vi "main.vi"() -> ()   [LabVIEW 2023]
uses:
  <vilib>/Utility/error.llb/DialogType.ctl
panel:
  in  "Stop":bool
  out "error out":errorcluster
  in  "error in (no error)":errorcluster
  out "Output":string
  in  "Commands":string
  in  "Execute":bool
  # "Note:\n    - SOURce:VOLTage:DC <voltage> \n    - SOURce:CURRent:DC <voltage>\n    - MEASure:VOLTage:DC ? \n    - MEASure:CURRent:DC ?"
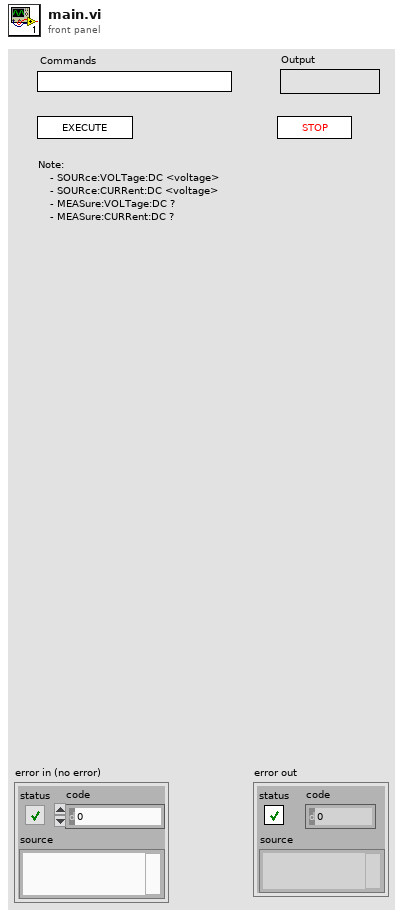
[diagram p1: front panel]
types:
  T1 = typedef "DialogType.ctl" = u16
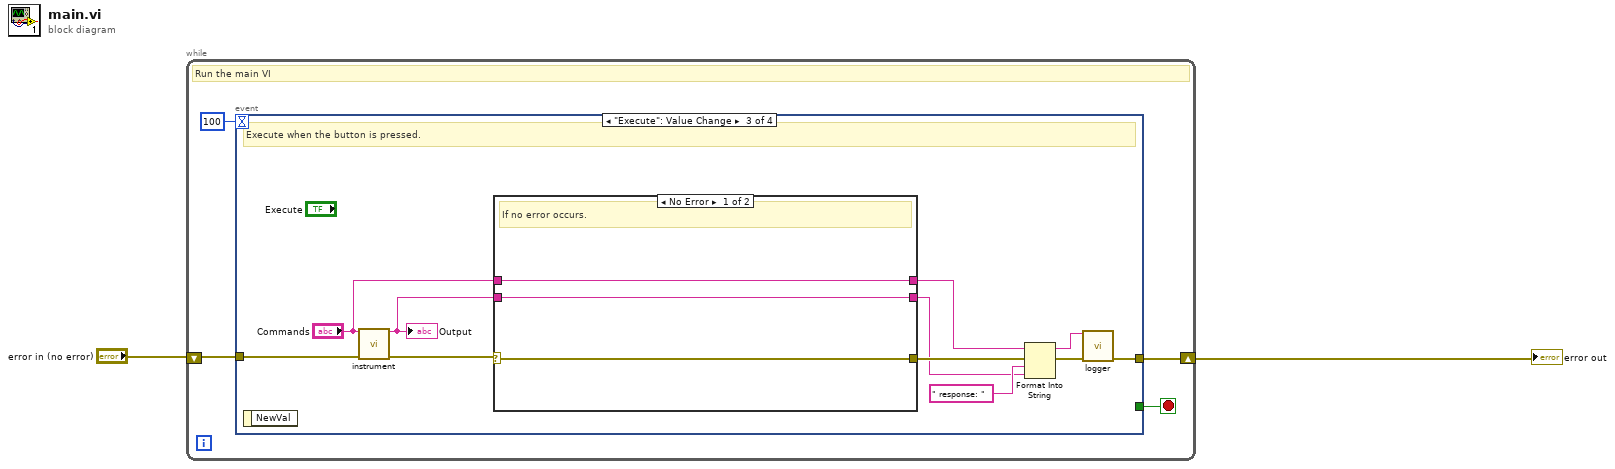
[diagram p0: block diagram]
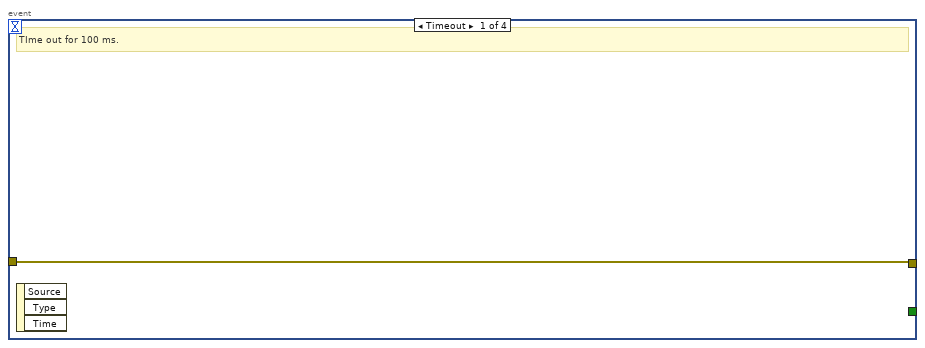
[diagram p2: hidden frame]
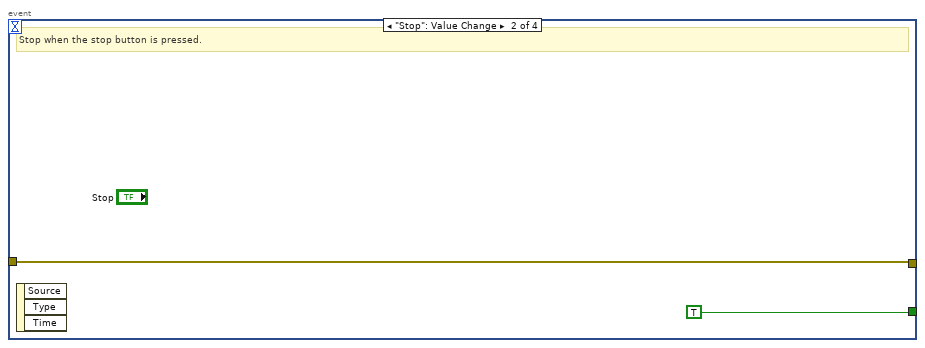
[diagram p3: hidden frame]
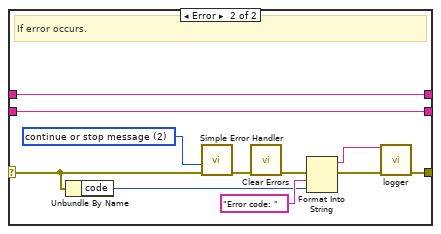
[diagram p4: hidden frame]
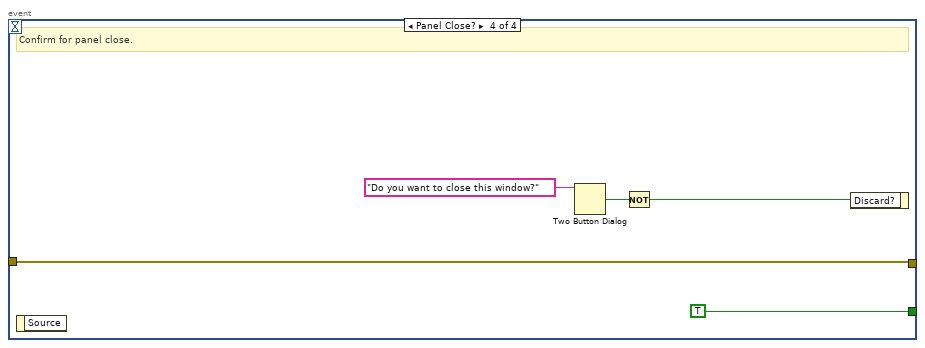
[diagram p5: hidden frame]
diagram:
  n1 = while {
    shift-right: [w4] -> w2
    shift-left: "error in (no error)" -> [w3]
    stop <- w5 stop-if-true
    # "Run the main VI"
    n2 = event shown="[2] \"Execute\": Value Change" {
      selector: _ -> [_ _ _ _]
      dyn-events: _ -> [_ _ _ _]
      timeout: 100 -> [_ _ _ _]
      tunnel: [_ TRUE _ TRUE] -> w5
      tunnel: [w7 w8 w16 w35] -> w4
      tunnel: w3 -> [w7 w8 w20 w35]
      event Timeout {
        # "TIme out for 100 ms."
        n3 = event-data() -> ()  [unwired: 1 in, 3 out]
      }
      event "Stop": Value Change {
        # "Stop when the stop button is pressed."
        n4 = event-data() -> ()  [unwired: 1 in, 3 out]
      }
      event "Execute": Value Change {
        # "Execute when the button is pressed."
        n5 = event-data() -> ()  [unwired: 1 in, 1 out]
        n6 = call "instrument.vi"("Commands"="Commands", "error in (no error)"=w20) -> ("Output"=w12:string, "error out"=w19:errorcluster)  [unwired: 12 in]
        "Output" <- w12
        n7 = case shown="No Error" w19 {
          selector: w19 -> [w23 w31]
          tunnel: [w23 w28] -> w15
          tunnel: "Commands" -> [w22 w25]
          tunnel: w12 -> [w21 w24]
          tunnel: [w22 w25] -> w11
          tunnel: [w21 w24] -> w10
          frame No Error {
            # "If no error occurs."
          }
          frame Error {
            w34 = T1 2 items=["no dialog", "OK message", "continue or stop message", "OK message + warnings", "continue/stop + warnings"] ("type of dialog (OK msg:1)")
            # "If error occurs."
            n8 = Unbundle By Name(w31) -> ("code"=w32:i32)
            n9 = call <vilib>:"Simple Error Handler.vi"("type of dialog (OK msg:1)"=w34, "error in (no error)"=w31) -> ("error out"=w29:errorcluster)  [unwired: 3 in, 4 out]
            n10 = call <vilib>:"Clear Errors.vi"("error in (no error)"=w29) -> ("error out"=w27:errorcluster)  [unwired: 5 in, 1 out]
            n11 = Format Into String(error in=w27, "Error code: ", w32) -> (resulting string=w30:string, error out=w26:errorcluster)  [unwired: 2 in]
            n12 = call "logger.vi"("Message"=w30, "error in"=w26) -> ("error out"=w28:errorcluster)  [unwired: 13 in]
          }
        }
        n13 = Format Into String(initial string=w11, error in=w15, " response: ", w10) -> (resulting string=w18:string, error out=w14:errorcluster)  [unwired: 1 in]
        n14 = call "logger.vi"("Message"=w18, "error in"=w14) -> ("error out"=w16:errorcluster)  [unwired: 13 in]
      }
      event Panel Close? {
        # "Confirm for panel close."
        n15 = event-data() -> ()  [unwired: 1 in, 1 out]
        n16 = Two Button Dialog(message="Do you want to close this window?") -> (T button?=w38:bool)  [unwired: 2 in]
        n17 = Not(x=w38) -> (.not. x?=w37:bool)
        n18 = event-data("Discard?"=w37) -> ()  [unwired: 1 in, 1 out]
      }
    }
  }
  "error out" <- w2
